vi "SERIAL_Initialize.vi"(1 "navX Device TypeDef":T1={"navX Interface Protocol"=enum."SPI", "navX Interface Protocol TypeDefs"={"SPIDevRef"={"DevStatus"={"status"=FALSE, "code"=0, "source"=""}, "Handle"=0, "Controller"=enum."Controller 1", "SPI Bus"=enum."SPI On-Board, CS0"}, "I2CDevRef"={"DevStatus"={"status"=FALSE, "code"=0, "source"=""}, "Controller"=enum."Controller 1", "Device Address"=0, "Handle"=0, "I2C Bus"=enum."Invalid"}, "SerialPortRef"={"DevStatus"={"status"=FALSE, "code"=0, "source"=""}, "Serial Port Name"=""}}, "navX System Information"={"Board Information"={"WhoAmI (50 | 0x32)"=0, "Board Revision"=0, "Firmware Major Version"=0, "Firmware Minor Version"=0, "NAVX_BOARD_CAPABILITY"={"OMNIMOUNT"=FALSE, "YAW_RESET"=FALSE, "VEL_AND_DISP"=FALSE}, "NAVX_BOARD_YAW_AXIS"={"BOARD_YAW_AXIS_UP"=FALSE, "BOARD_YAW_AXIS"=0}}, "Status"={"Update Rate Hz"=0, "Accelerometer Full-Scale Range"=0, "Gyro Full-Scale Range"=0, "NAVX_OP_STATUS"=0, "NAVX_CAL_STATUS"=0, "NAVX_SELFTEST_STATUS"=0, "NAVX_SENSOR_STATUS"={"MOVING"=FALSE, "YAW_STABLE"=FALSE, "MAG_DISTURBANCE"=FALSE, "ALTITUDE_VALID"=FALSE, "SEALEVEL_PRESS_SET"=FALSE, "FUSED_HEADING_VALID"=FALSE}}, "Offsets"={"Yaw"=0.0, "Quat W"=0.0, "Quat X"=0.0, "Quat Y"=0.0, "Quat Z"=0.0}, "LastSampleTimestamp"=0.0, "LastSampleValid"=FALSE}, "navX Common Information"={"Update Rate (4Hz-60Hz)"=50, "refnum name"="", "error"={"status"=FALSE, "code"=0, "source"=""}, "LastFPGATimestamp"=0.0, "Reboot Detected"=FALSE}, "Serial Protocol Extra"={"Loop VI Refnum"=refnum, "Nav6Mode (YPR)"=enum."Raw"}} {"navX Common Information"."Update Rate (4Hz-60Hz)" min=4 max=60 step=1; "navX System Information"."Status"."NAVX_OP_STATUS" items=["INITIALIZING", "SELFTEST_IN_PROGRESS", "ERROR", "IMU_AUTOCAL_IN_PROGRESS", "NORMAL"]; "navX System Information"."Status"."NAVX_CAL_STATUS" items=["IMU_CAL_STATE_MASK"=3, "IMU_CAL_INPROGRESS"=0, "IMU_CAL_ACCUMULATE"=1, "IMU_CAL_COMPLETE"=2, "MAG_CAL_COMPLETE"=4, "BARO_CAL_COMPLETE"=8]; "navX System Information"."Status"."NAVX_SELFTEST_STATUS" items=["COMPLETE"=80, "GYRO_PASSED"=1, "ACCEL_PASSED"=2, "MAG_PASSED"=4, "BARO_PASSED"=8]; "navX Interface Protocol TypeDefs"."I2CDevRef"."Device Address" format="%.0x"}) -> (0 "navX Device TypeDef":T1={"navX Interface Protocol"=enum."SPI", "navX Interface Protocol TypeDefs"={"SPIDevRef"={"DevStatus"={"status"=FALSE, "code"=0, "source"=""}, "Handle"=0, "Controller"=enum."Controller 1", "SPI Bus"=enum."SPI On-Board, CS0"}, "I2CDevRef"={"DevStatus"={"status"=FALSE, "code"=0, "source"=""}, "Controller"=enum."Controller 1", "Device Address"=0, "Handle"=0, "I2C Bus"=enum."Invalid"}, "SerialPortRef"={"DevStatus"={"status"=FALSE, "code"=0, "source"=""}, "Serial Port Name"=""}}, "navX System Information"={"Board Information"={"WhoAmI (50 | 0x32)"=0, "Board Revision"=0, "Firmware Major Version"=0, "Firmware Minor Version"=0, "NAVX_BOARD_CAPABILITY"={"OMNIMOUNT"=FALSE, "YAW_RESET"=FALSE, "VEL_AND_DISP"=FALSE}, "NAVX_BOARD_YAW_AXIS"={"BOARD_YAW_AXIS_UP"=FALSE, "BOARD_YAW_AXIS"=0}}, "Status"={"Update Rate Hz"=0, "Accelerometer Full-Scale Range"=0, "Gyro Full-Scale Range"=0, "NAVX_OP_STATUS"=0, "NAVX_CAL_STATUS"=0, "NAVX_SELFTEST_STATUS"=0, "NAVX_SENSOR_STATUS"={"MOVING"=FALSE, "YAW_STABLE"=FALSE, "MAG_DISTURBANCE"=FALSE, "ALTITUDE_VALID"=FALSE, "SEALEVEL_PRESS_SET"=FALSE, "FUSED_HEADING_VALID"=FALSE}}, "Offsets"={"Yaw"=0.0, "Quat W"=0.0, "Quat X"=0.0, "Quat Y"=0.0, "Quat Z"=0.0}, "LastSampleTimestamp"=0.0, "LastSampleValid"=FALSE}, "navX Common Information"={"Update Rate (4Hz-60Hz)"=50, "refnum name"="", "error"={"status"=FALSE, "code"=0, "source"=""}, "LastFPGATimestamp"=0.0, "Reboot Detected"=FALSE}, "Serial Protocol Extra"={"Loop VI Refnum"=refnum, "Nav6Mode (YPR)"=enum."Raw"}} {"navX Common Information"."Update Rate (4Hz-60Hz)" min=4 max=60 step=1; "navX System Information"."Status"."NAVX_OP_STATUS" items=["INITIALIZING", "SELFTEST_IN_PROGRESS", "ERROR", "IMU_AUTOCAL_IN_PROGRESS", "NORMAL"]; "navX System Information"."Status"."NAVX_CAL_STATUS" items=["IMU_CAL_STATE_MASK"=3, "IMU_CAL_INPROGRESS"=0, "IMU_CAL_ACCUMULATE"=1, "IMU_CAL_COMPLETE"=2, "MAG_CAL_COMPLETE"=4, "BARO_CAL_COMPLETE"=8]; "navX System Information"."Status"."NAVX_SELFTEST_STATUS" items=["COMPLETE"=80, "GYRO_PASSED"=1, "ACCEL_PASSED"=2, "MAG_PASSED"=4, "BARO_PASSED"=8]; "navX Interface Protocol TypeDefs"."I2CDevRef"."Device Address" format="%.0x"})   [LabVIEW 2014, in "navX-MXP IMU.lvlib"]
uses:
  navX-MXP IMU.lvlib
  COMMON/TypeDefs/navX Device TypeDef.ctl
  COMMON/TypeDefs/Value TypeDefs/navX Interface Protocol.ctl
  <vilib>/Rock Robotics/WPI/SPI/WPI_SPIDevRef.ctl
  <vilib>/Rock Robotics/SystemInterfaces/Typedef/FPGA_TypedefDigitalModule.ctl
  <vilib>/Rock Robotics/SystemInterfaces/spilib/spi_bus.ctl
  <vilib>/Rock Robotics/WPI/I2C/WPI_I2CDevRef.ctl
  <vilib>/Rock Robotics/SystemInterfaces/i2clib/i2c_bus.ctl
  <vilib>/Rock Robotics/WPI/SerialPort/WPI_SerialPortRef.ctl
  COMMON/TypeDefs/Data TypeDefs/navX Board Information.ctl
  COMMON/TypeDefs/Value TypeDefs/navX NAVX_BOARD_CAPABILITY.ctl
  COMMON/TypeDefs/Value TypeDefs/navX NAVX_BOARD_YAW_AXIS.ctl
  COMMON/TypeDefs/Data TypeDefs/navX Status Data.ctl
  COMMON/TypeDefs/Value TypeDefs/navX NAVX_OP_STATUS.ctl
  COMMON/TypeDefs/Value TypeDefs/navX NAVX_CAL_STATUS.ctl
  COMMON/TypeDefs/Value TypeDefs/navX NAVX_SELFTEST_STATUS.ctl
  COMMON/TypeDefs/Value TypeDefs/navX NAVX_SENSOR_STATUS.ctl
  COMMON/TypeDefs/Data TypeDefs/navX Offsets Data.ctl
  COMMON/TypeDefs/Value TypeDefs/navX Update Rate.ctl
  COMMON/TypeDefs/Value TypeDefs/navX Serial Mode.ctl
  COMMON/TypeDefs/Value TypeDefs/navX Device Registers.ctl
  COMMON/TypeDefs/Value TypeDefs/navX NAVX_CAPABILITY_FLAGS.ctl
  <vilib>/Rock Robotics/SystemInterfaces/Utilities/FPGA_UtilitiesRead LocalTime.vi
  COMMON/Util/DataConvert/navX-to-LabVIEW/DecodeRatio.vi
  COMMON/Util/DataConvert/navX-to-LabVIEW/DecodeSignedHundredths.vi
  COMMON/Util/DataConvert/navX-to-LabVIEW/DecodeUInt16.vi
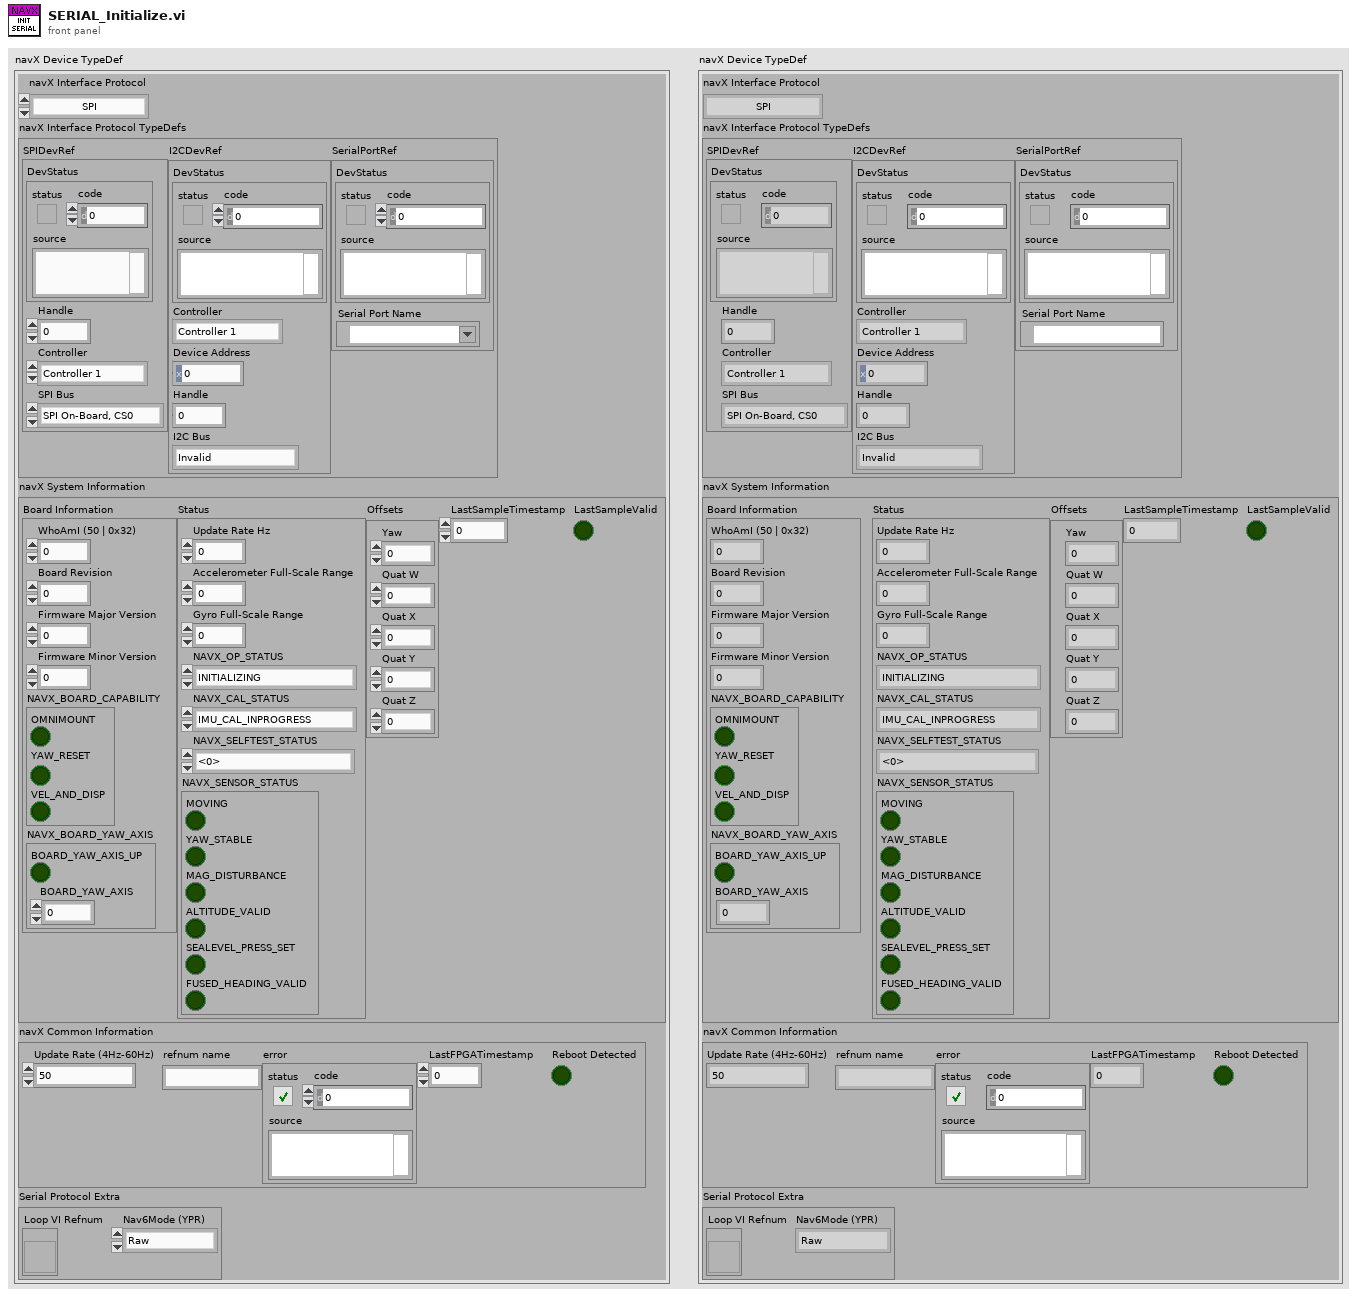
[diagram p1: front panel]
types:
  T1 = typedef "navX-MXP IMU.lvlib/navX Device TypeDef.ctl" = cluster{"navX Interface Protocol":T2, "navX Interface Protocol TypeDefs":cluster{"SPIDevRef":T3, "I2CDevRef":T6, "SerialPortRef":T8}, "navX System Information":cluster{"Board Information":T9, "Status":T12, "Offsets":T17, "LastSampleTimestamp":dbl, "LastSampleValid":bool}, "navX Common Information":cluster{"Update Rate (4Hz-60Hz)":T18, "refnum name":string, "error":errorcluster, "LastFPGATimestamp":dbl, "Reboot Detected":bool}, "Serial Protocol Extra":cluster{"Loop VI Refnum":refnum<vi>, "Nav6Mode (YPR)":T19}}
  T2 = typedef "navX-MXP IMU.lvlib/navX Interface Protocol.ctl" = enum16{"SPI", "I2C", "SERIAL"}
  T3 = typedef "WPI_SPIDevRef.ctl" = cluster{"DevStatus":errorcluster, "Handle":i32, "Controller":T4, "SPI Bus":T5}
  T4 = typedef "FPGA_TypedefDigitalModule.ctl" = enum16{"Controller 1"}
  T5 = typedef "spi_bus.ctl" = enum16{"SPI On-Board, CS0", "SPI On-Board, CS1", "SPI On-Board, CS2", "SPI On-Board, CS3", "SPI MXP", "Invalid"}
  T6 = typedef "WPI_I2CDevRef.ctl" = cluster{"DevStatus":errorcluster, "Controller":T4, "Device Address":u8, "Handle":i32, "I2C Bus":T7}
  T7 = typedef "i2c_bus.ctl" = enum16{"I2C On-Board", "I2C MXP", "Invalid"}
  T8 = typedef "WPI_SerialPortRef.ctl" = cluster{"DevStatus":errorcluster, "Serial Port Name":refnum<visa-resource-name>}
  T9 = typedef "navX-MXP IMU.lvlib/navX Board Information.ctl" = cluster{"WhoAmI (50 | 0x32)":u8, "Board Revision":u8, "Firmware Major Version":u8, "Firmware Minor Version":u8, "NAVX_BOARD_CAPABILITY":T10, "NAVX_BOARD_YAW_AXIS":T11}
  T10 = typedef "navX-MXP IMU.lvlib/navX NAVX_BOARD_CAPABILITY.ctl" = cluster{"OMNIMOUNT":bool, "YAW_RESET":bool, "VEL_AND_DISP":bool}
  T11 = typedef "navX-MXP IMU.lvlib/navX NAVX_BOARD_YAW_AXIS.ctl" = cluster{"BOARD_YAW_AXIS_UP":bool, "BOARD_YAW_AXIS":u8}
  T12 = typedef "navX-MXP IMU.lvlib/navX Status Data.ctl" = cluster{"Update Rate Hz":u8, "Accelerometer Full-Scale Range":u8, "Gyro Full-Scale Range":u16, "NAVX_OP_STATUS":T13, "NAVX_CAL_STATUS":T14, "NAVX_SELFTEST_STATUS":T15, "NAVX_SENSOR_STATUS":T16}
  T13 = typedef "navX-MXP IMU.lvlib/navX NAVX_OP_STATUS.ctl" = u8
  T14 = typedef "navX-MXP IMU.lvlib/navX NAVX_CAL_STATUS.ctl" = u8
  T15 = typedef "navX-MXP IMU.lvlib/navX NAVX_SELFTEST_STATUS.ctl" = u8
  T16 = typedef "navX-MXP IMU.lvlib/navX NAVX_SENSOR_STATUS.ctl" = cluster{"MOVING":bool, "YAW_STABLE":bool, "MAG_DISTURBANCE":bool, "ALTITUDE_VALID":bool, "SEALEVEL_PRESS_SET":bool, "FUSED_HEADING_VALID":bool}
  T17 = typedef "navX-MXP IMU.lvlib/navX Offsets Data.ctl" = cluster{"Yaw":dbl, "Quat W":dbl, "Quat X":dbl, "Quat Y":dbl, "Quat Z":dbl}
  T18 = typedef "navX-MXP IMU.lvlib/navX Update Rate.ctl" = u8
  T19 = typedef "navX-MXP IMU.lvlib/navX Serial Mode.ctl" = enum16{"Raw", "Processed"}
  T20 = typedef "navX-MXP IMU.lvlib/navX Device Registers.ctl" = u8
  T21 = typedef "navX-MXP IMU.lvlib/navX NAVX_CAPABILITY_FLAGS.ctl" = u8
  T22 = cluster{"[0]":dbl, "[1]":dbl, "[2]":dbl, "[3]":dbl, "[4]":dbl}
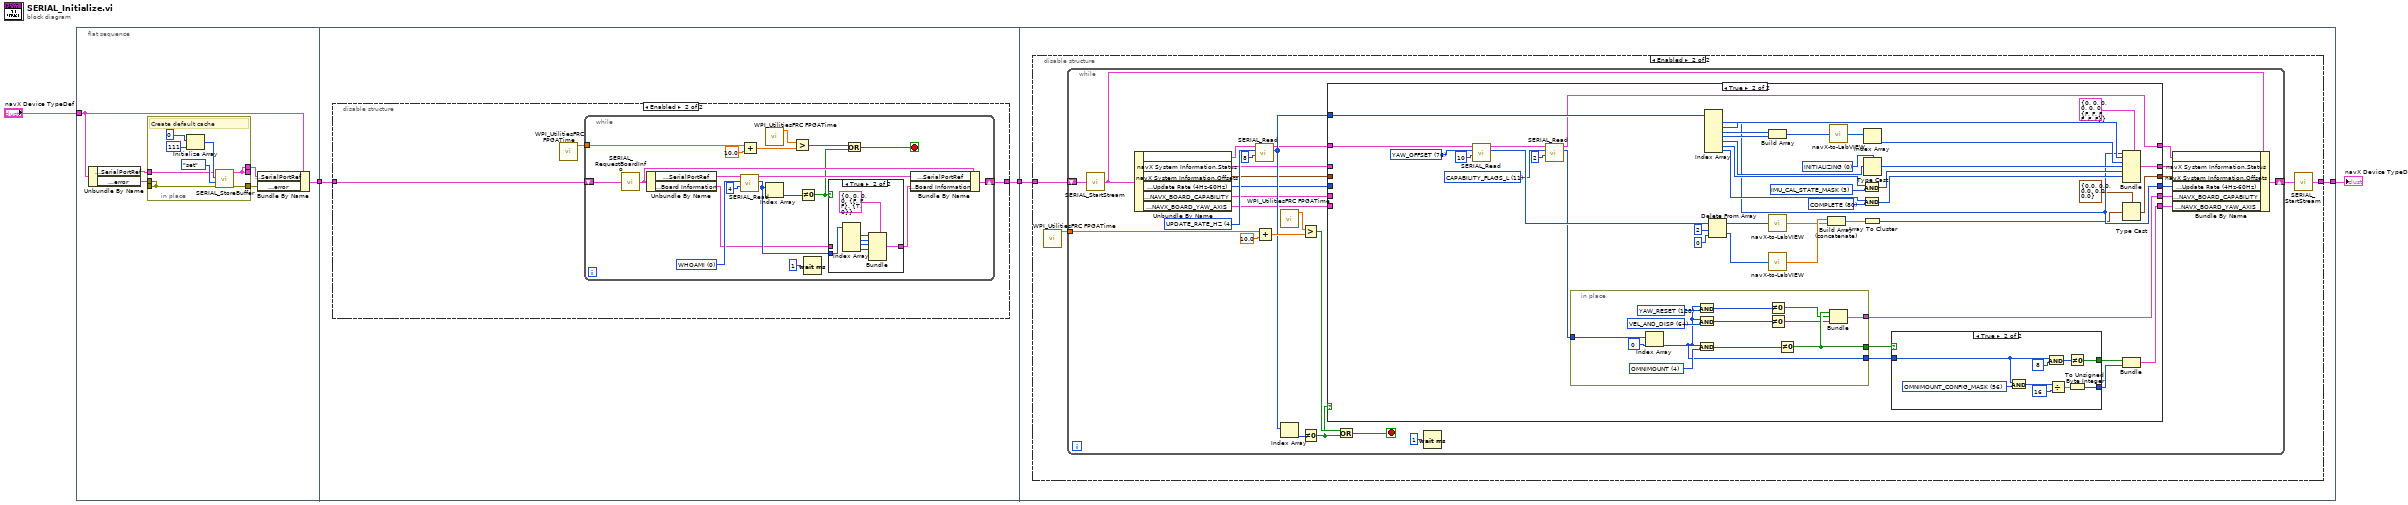
[diagram p0: block diagram]
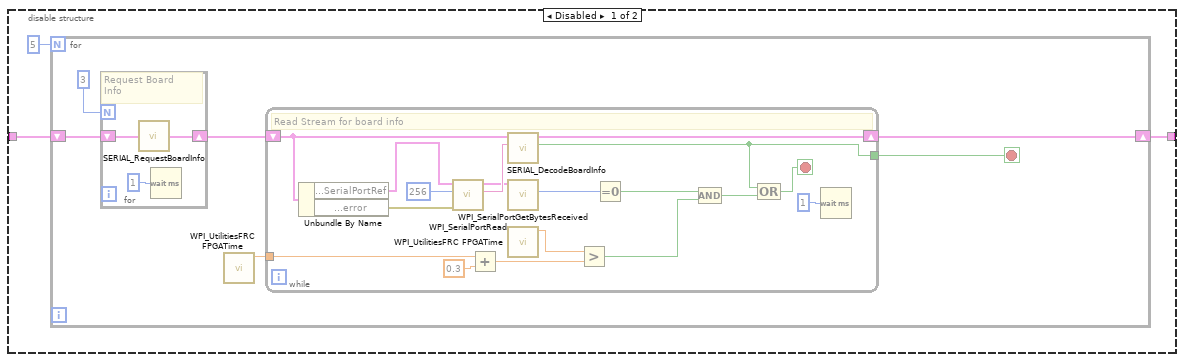
[diagram p2: hidden frame]
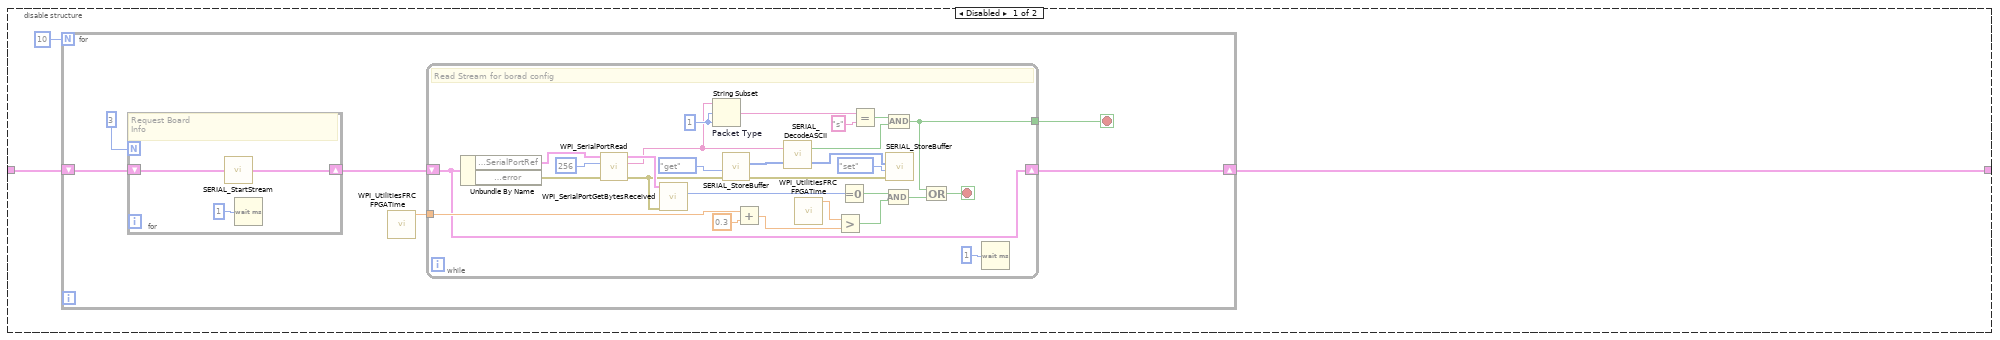
[diagram p4: hidden frame]
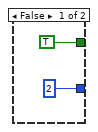
[diagram p6: hidden frame]
diagram:
  n1 = flat-sequence {
    tunnel: "navX Device TypeDef" -> [w6]
    tunnel: [w5] -> w1
    tunnel: [w20] -> w2
    tunnel: w1 -> [w19]
    tunnel: [w81] -> w4
    tunnel: w2 -> [w82]
    frame #0 {
      n2 = Unbundle By Name(w6) -> ("navX Interface Protocol TypeDefs.SerialPortRef"=w10:T8, "navX Common Information.error"=w9:errorcluster)
      n3 = in-place {
        in-place-border: w10 -> [w14]
        in-place-border: [w12] -> _
        in-place-border: [w13] -> w8
        in-place-border: [w11] -> _
        in-place-border: w9 -> [w12]
        in-place-border: [w11] -> w7
        # "Create default cache"
        n4 = Initialize Array(u8 0 ("Received Data"), u8 111 ("hex")) -> (w15:u8[])
        n5 = call "SERIAL_StoreBuffer.vi"("error in (no error)"=w12, "Access Type"=enum16{"set", "get", "delete"}."set", "navX Data"=w15, "SerialPortRef"=w14) -> ("error out"=w13:errorcluster, "SerialPortRef"=w11:T8)  [unwired: 5 in, 1 out]
      }
      n6 = Bundle By Name(cluster=w6, "navX Interface Protocol TypeDefs.SerialPortRef"=w7, "navX Common Information.error"=w8) -> (w5:T1)
    }
    frame #1 {
      n7 = disable-structure shown="Enabled" {
        disable-tunnel: [w23 w52] -> w20
        disable-tunnel: w19 -> [w22 w53]
        frame Disabled {
          n8 = for {
            N: 5 -> [_]
            shift-right: [w25] -> w23
            shift-left: w22 -> [w27]
            stop <- w24 stop-if-true
            n9 = for {
              N: 3 -> [_]
              shift-right: [w31] -> w28
              shift-left: w27 -> [w32]
              # "Request Board\nInfo"
              n10 = call "SERIAL_RequestBoardInfo.vi"("navX Device TypeDef"=w32) -> ("navX Device TypeDef"=w31:T1)
              n11 = Wait (ms)(milliseconds to wait=u32 1) -> ()  [unwired: 1 out]
            }
            n12 = call <vilib>:"WPI_UtilitiesFRC FPGATime.vi"() -> ("FPGA Time"=w26:dbl)  [unwired: 10 in, 1 out]
            n13 = while {
              tunnel: w26 -> [w50]
              shift-right: [w35] -> w25
              shift-left: w28 -> [w41]
              tunnel: [w34] -> w24
              stop <- w36 stop-if-true
              # "Read Stream for board info"
              n14 = Unbundle By Name(w41) -> ("navX Interface Protocol TypeDefs.SerialPortRef"=w43:T8, "navX Common Information.error"=w44:errorcluster)
              n15 = call <vilib>:"WPI_SerialPortRead.vi"("error in (no error)"=w44, "Num Bytes to Read"=u32 256, "SerialPortRef"=w43) -> ("Buffer"=w40:string, "SerialPortRef"=w39:T8)  [unwired: 6 in, 1 out]
              n16 = Add(x=w50, y=0.3) -> (x+y=w47:dbl)
              n17 = call "SERIAL_DecodeBoardInfo.vi"("Buffer"=w40, "navX Device TypeDef"=w41) -> ("Valid?"=w34:bool, "navX Device TypeDef"=w35:T1)  [unwired: 8 in]
              n18 = call <vilib>:"WPI_SerialPortGetBytesReceived.vi"("SerialPortRef"=w39) -> ("Bytes at Port"=w38:u32)  [unwired: 8 in, 2 out]
              n19 = call <vilib>:"WPI_UtilitiesFRC FPGATime.vi"() -> ("FPGA Time"=w48:dbl)  [unwired: 10 in, 1 out]
              n20 = Greater?(x=w48, y=w47) -> (0:w45:bool)
              n21 = Equal To 0?(x=w38) -> (x = 0?=w37:bool)
              n22 = Compound Arithmetic op=AND(w37, w45) -> (w46:bool)
              n23 = Compound Arithmetic op=OR(w34, w46) -> (w36:bool)
              n24 = Wait (ms)(milliseconds to wait=u32 1) -> ()  [unwired: 1 out]
            }
          }
        }
        frame Enabled {
          n25 = call <vilib>:"WPI_UtilitiesFRC FPGATime.vi"() -> ("FPGA Time"=w51:dbl)  [unwired: 10 in, 1 out]
          n26 = while {
            shift-right: [w60] -> w52
            shift-left: w53 -> [w72]
            tunnel: w51 -> [w67]
            stop <- w66 stop-if-true
            w58 = T20 0 items=["WHOAMI"=0, "HW_REV"=1, "FW_VER_MAJOR"=2, "FW_VER_MINOR"=3, "UPDATE_RATE_HZ"=4, "ACCEL_FSR_G"=5, "GYRO_FSR_DPS"=6, "OP_STATUS"=8, "CAL_STATUS"=9, "SELFTEST_STATUS"=10, "CAPABILITY_FLAGS_L"=11, "CAPABILITY_FLAGS_H"=12, "SENSOR_STATUS"=16, "TIMESTAMP"=18, "YAW"=22, "PITCH"=24, "ROLL"=26, "HEADING"=28, "FUSED_HEADING"=30, "ALTITUDE_I"=32, "ALTITUDE_D"=34, "LINERA_ACC_X"=36, "LINERA_ACC_Y"=38, "LINERA_ACC_Z"=40, "QUAT_W"=42, "QUAT_X"=44, "QUAT_Y"=46, "QUAT_Z"=48, "MPU_TEMP_C"=50, "GYRO_X"=52, "GYRO_Y"=54, "GYRO_Z"=56, "ACC_X"=58, "ACC_Y"=60, "ACC_Z"=62, "MAG_X"=64, "MAG_Y"=66, "MAG_Z"=68, "PRESSURE_I"=70, "PRESSURE_D"=72, "PRESSURE_TEMP"=74, "YAW_OFFSET"=76, "QUAT_OFFSET_W"=78, "QUAT_OFFSET_X"=80, "QUAT_OFFSET_Y"=82, "QUAT_OFFSET_Z"=84, "INTEGRATION_CONTROL"=86, "VELOCITY_X"=88, "VELOCITY_Y"=92, "VELOCITY_Z"=96, "DISPLACMENT_X"=100, "DISPLACMENT_Y"=104, "DISPLACEMENT_Z"=108] ("Device Register")
            n27 = call "SERIAL_RequestBoardInfo.vi"("navX Device TypeDef"=w72) -> ("navX Device TypeDef"=w64:T1)
            n28 = Unbundle By Name(w64) -> ("navX Interface Protocol TypeDefs.SerialPortRef"=w63:T8, "navX System Information.Board Information"=w54:T9)
            n29 = call "SERIAL_Read.vi"("Read Size"=u8 4, "Device Register"=w58, "SerialPortRef"=w63) -> ("navX Data"=w57:u8[], "SerialPortRef"=w62:T8)  [unwired: 6 in, 1 out]
            n30 = Add(x=w67, y=10.0) -> (x+y=w69:dbl)
            n31 = call <vilib>:"WPI_UtilitiesFRC FPGATime.vi"() -> ("FPGA Time"=w70:dbl)  [unwired: 10 in, 1 out]
            n32 = Index Array(array=w57) -> (element=w61:u8)  [unwired: 1 in]
            n33 = Greater?(x=w70, y=w69) -> (0:w65:bool)
            n34 = Not Equal To 0?(x=w61) -> (x != 0?=w55:bool)
            n35 = Wait (ms)(milliseconds to wait=u32 1) -> ()  [unwired: 1 out]
            n36 = case shown="True" w55 {
              tunnel: w57 -> [_ w80]
              tunnel: [w73 w79] -> w56
              tunnel: w54 -> [w73 _]
              frame False {
              }
              frame True {
                n37 = Index Array(array=w80) -> (element #1=w77:u8, element #2=w76:u8, element #3=w75:u8, element #4=w74:u8)  [unwired: 4 in]
                n38 = Bundle(cluster=T9 {"WhoAmI (50 | 0x32)"=0, "Board Revision"=0, "Firmware Major Version"=0, "Firmware Minor Version"=0, "NAVX_BOARD_CAPABILITY"={"OMNIMOUNT"=FALSE, "YAW_RESET"=FALSE, "VEL_AND_DISP"=FALSE}, "NAVX_BOARD_YAW_AXIS"={"BOARD_YAW_AXIS_UP"=TRUE, "BOARD_YAW_AXIS"=0}} ("Board Information"), "WhoAmI (50 | 0x32)"=w77, "Board Revision"=w76, "Firmware Major Version"=w75, "Firmware Minor Version"=w74) -> (w79:T9)  [unwired: 2 in]
              }
            }
            n39 = Or(x=w65, y=w55) -> (x .or. y?=w66:bool)
            n40 = Bundle By Name(cluster=w64, "navX Interface Protocol TypeDefs.SerialPortRef"=w62, "navX System Information.Board Information"=w56) -> (w60:T1)
          }
        }
      }
    }
    frame #2 {
      n41 = disable-structure shown="Enabled" {
        disable-tunnel: w82 -> [w84 w126]
        disable-tunnel: [w83 w123] -> w81
        frame Disabled {
          n42 = for {
            N: 10 -> [_]
            shift-right: [w87] -> w83
            shift-left: w84 -> [w89]
            stop <- w86 stop-if-true
            n43 = for {
              N: 3 -> [_]
              shift-right: [w92] -> w90
              shift-left: w89 -> [w93]
              # "Request Board\nInfo"
              n44 = call "SERIAL_StartStream.vi"("navX Device TypeDef"=w93) -> ("navX Device TypeDef"=w92:T1)
              n45 = Wait (ms)(milliseconds to wait=u32 1) -> ()  [unwired: 1 out]
            }
            n46 = call <vilib>:"WPI_UtilitiesFRC FPGATime.vi"() -> ("FPGA Time"=w88:dbl)  [unwired: 10 in, 1 out]
            n47 = while {
              tunnel: w88 -> [w122]
              shift-right: [w108] -> w87
              shift-left: w90 -> [w108]
              tunnel: [w97] -> w86
              stop <- w110 stop-if-true
              w105 = 1 ("offset (0)")
              # "Read Stream for borad config"
              n48 = Unbundle By Name(w108) -> ("navX Interface Protocol TypeDefs.SerialPortRef"=w115:T8, "navX Common Information.error"=w116:errorcluster)
              n49 = call <vilib>:"WPI_SerialPortRead.vi"("error in (no error)"=w116, "Num Bytes to Read"=u32 256, "SerialPortRef"=w115) -> ("error out"=w95:errorcluster, "Buffer"=w104:string, "SerialPortRef"=w113:T8)  [unwired: 6 in]
              n50 = call <vilib>:"WPI_SerialPortGetBytesReceived.vi"("error in (no error)"=w95, "SerialPortRef"=w113) -> ("Bytes at Port"=w112:u32)  [unwired: 7 in, 2 out]
              n51 = String Subset "Packet Type"(string=w104, offset (0)=w105, length (rest)=w105) -> (substring=w103:string)
              n52 = call "SERIAL_StoreBuffer.vi"("error in (no error)"=w95, "Access Type"=enum16{"set", "get", "delete"}."get") -> ("error out"=w96:errorcluster, "navX Data"=w107:u8[])  [unwired: 7 in, 1 out]
              n53 = Add(x=w122, y=0.3) -> (x+y=w119:dbl)
              n54 = call "SERIAL_DecodeASCII.vi"("navX Data"=w107, "Buffer"=w104) -> ("navX Data"=w100:u8[], "Valid?"=w98:bool)
              n55 = call <vilib>:"WPI_UtilitiesFRC FPGATime.vi"() -> ("FPGA Time"=w120:dbl)  [unwired: 10 in, 1 out]
              n56 = Greater?(x=w120, y=w119) -> (0:w117:bool)
              n57 = Equal To 0?(x=w112) -> (x = 0?=w111:bool)
              n58 = Equal?(x=w103, y="s") -> (x = y?=w99:bool)
              n59 = call "SERIAL_StoreBuffer.vi"("error in (no error)"=w96, "Access Type"=enum16{"set", "get", "delete"}."set", "navX Data"=w100) -> ()  [unwired: 6 in, 3 out]
              n60 = Compound Arithmetic op=AND(w111, w117) -> (w118:bool)
              n61 = Compound Arithmetic op=AND(w99, w98) -> (w97:bool)
              n62 = Compound Arithmetic op=OR(w97, w118) -> (w110:bool)
              n63 = Wait (ms)(milliseconds to wait=u32 1) -> ()  [unwired: 1 out]
            }
          }
        }
        frame Enabled {
          n64 = call <vilib>:"WPI_UtilitiesFRC FPGATime.vi"() -> ("FPGA Time"=w125:dbl)  [unwired: 10 in, 1 out]
          n65 = while {
            shift-right: [w151] -> w124
            shift-left: w126 -> [w153]
            tunnel: w125 -> [w146]
            stop <- w144 stop-if-true
            w143 = T20 4 items=["WHOAMI"=0, "HW_REV"=1, "FW_VER_MAJOR"=2, "FW_VER_MINOR"=3, "UPDATE_RATE_HZ"=4, "ACCEL_FSR_G"=5, "GYRO_FSR_DPS"=6, "OP_STATUS"=8, "CAL_STATUS"=9, "SELFTEST_STATUS"=10, "CAPABILITY_FLAGS_L"=11, "CAPABILITY_FLAGS_H"=12, "SENSOR_STATUS"=16, "TIMESTAMP"=18, "YAW"=22, "PITCH"=24, "ROLL"=26, "HEADING"=28, "FUSED_HEADING"=30, "ALTITUDE_I"=32, "ALTITUDE_D"=34, "LINERA_ACC_X"=36, "LINERA_ACC_Y"=38, "LINERA_ACC_Z"=40, "QUAT_W"=42, "QUAT_X"=44, "QUAT_Y"=46, "QUAT_Z"=48, "MPU_TEMP_C"=50, "GYRO_X"=52, "GYRO_Y"=54, "GYRO_Z"=56, "ACC_X"=58, "ACC_Y"=60, "ACC_Z"=62, "MAG_X"=64, "MAG_Y"=66, "MAG_Z"=68, "PRESSURE_I"=70, "PRESSURE_D"=72, "PRESSURE_TEMP"=74, "YAW_OFFSET"=76, "QUAT_OFFSET_W"=78, "QUAT_OFFSET_X"=80, "QUAT_OFFSET_Y"=82, "QUAT_OFFSET_Z"=84, "INTEGRATION_CONTROL"=86, "VELOCITY_X"=88, "VELOCITY_Y"=92, "VELOCITY_Z"=96, "DISPLACMENT_X"=100, "DISPLACMENT_Y"=104, "DISPLACEMENT_Z"=108] ("Device Register")
            n66 = call "SERIAL_StartStream.vi"("navX Device TypeDef"=w153) -> ("navX Device TypeDef"=w152:T1)
            n67 = Unbundle By Name(w152) -> ("navX Interface Protocol TypeDefs.SerialPortRef"=w150:T8, "navX System Information.Status"=w138:T12, "navX System Information.Offsets"=w136:T17, "navX Common Information.Update Rate (4Hz-60Hz)"=w133:T18, "navX System Information.Board Information.NAVX_BOARD_CAPABILITY"=w128:T10, "navX System Information.Board Information.NAVX_BOARD_YAW_AXIS"=w127:T11)
            n68 = call "SERIAL_Read.vi"("Read Size"=u8 8, "Device Register"=w143, "SerialPortRef"=w150) -> ("navX Data"=w139:u8[], "SerialPortRef"=w132:T8)  [unwired: 6 in, 1 out]
            n69 = Add(x=w146, y=10.0) -> (x+y=w148:dbl)
            n70 = call <vilib>:"WPI_UtilitiesFRC FPGATime.vi"() -> ("FPGA Time"=w147:dbl)  [unwired: 10 in, 1 out]
            n71 = Index Array(array=w139) -> (element=w141:u8)  [unwired: 1 in]
            n72 = Greater?(x=w147, y=w148) -> (0:w149:bool)
            n73 = Not Equal To 0?(x=w141) -> (x != 0?=w140:bool)
            n74 = case shown="True" w140 {
              tunnel: w139 -> [_ w204]
              tunnel: [w160 w187] -> w137
              tunnel: w138 -> [w160 _]
              tunnel: w136 -> [w159 _]
              tunnel: [w159 w173] -> w135
              tunnel: [w158 w186] -> w134
              tunnel: w133 -> [w158 _]
              tunnel: w132 -> [w157 w167]
              tunnel: [w157 w165] -> w131
              tunnel: [w155 w162] -> w130
              tunnel: [w156 w161] -> w129
              tunnel: w128 -> [w156 _]
              tunnel: w127 -> [w155 _]
              frame False {
              }
              frame True {
                w172 = T20 11 items=["WHOAMI"=0, "HW_REV"=1, "FW_VER_MAJOR"=2, "FW_VER_MINOR"=3, "UPDATE_RATE_HZ"=4, "ACCEL_FSR_G"=5, "GYRO_FSR_DPS"=6, "OP_STATUS"=8, "CAL_STATUS"=9, "SELFTEST_STATUS"=10, "CAPABILITY_FLAGS_L"=11, "CAPABILITY_FLAGS_H"=12, "SENSOR_STATUS"=16, "TIMESTAMP"=18, "YAW"=22, "PITCH"=24, "ROLL"=26, "HEADING"=28, "FUSED_HEADING"=30, "ALTITUDE_I"=32, "ALTITUDE_D"=34, "LINERA_ACC_X"=36, "LINERA_ACC_Y"=38, "LINERA_ACC_Z"=40, "QUAT_W"=42, "QUAT_X"=44, "QUAT_Y"=46, "QUAT_Z"=48, "MPU_TEMP_C"=50, "GYRO_X"=52, "GYRO_Y"=54, "GYRO_Z"=56, "ACC_X"=58, "ACC_Y"=60, "ACC_Z"=62, "MAG_X"=64, "MAG_Y"=66, "MAG_Z"=68, "PRESSURE_I"=70, "PRESSURE_D"=72, "PRESSURE_TEMP"=74, "YAW_OFFSET"=76, "QUAT_OFFSET_W"=78, "QUAT_OFFSET_X"=80, "QUAT_OFFSET_Y"=82, "QUAT_OFFSET_Z"=84, "INTEGRATION_CONTROL"=86, "VELOCITY_X"=88, "VELOCITY_Y"=92, "VELOCITY_Z"=96, "DISPLACMENT_X"=100, "DISPLACMENT_Y"=104, "DISPLACEMENT_Z"=108] ("Device Register")
                w184 = T20 76 items=["WHOAMI"=0, "HW_REV"=1, "FW_VER_MAJOR"=2, "FW_VER_MINOR"=3, "UPDATE_RATE_HZ"=4, "ACCEL_FSR_G"=5, "GYRO_FSR_DPS"=6, "OP_STATUS"=8, "CAL_STATUS"=9, "SELFTEST_STATUS"=10, "CAPABILITY_FLAGS_L"=11, "CAPABILITY_FLAGS_H"=12, "SENSOR_STATUS"=16, "TIMESTAMP"=18, "YAW"=22, "PITCH"=24, "ROLL"=26, "HEADING"=28, "FUSED_HEADING"=30, "ALTITUDE_I"=32, "ALTITUDE_D"=34, "LINERA_ACC_X"=36, "LINERA_ACC_Y"=38, "LINERA_ACC_Z"=40, "QUAT_W"=42, "QUAT_X"=44, "QUAT_Y"=46, "QUAT_Z"=48, "MPU_TEMP_C"=50, "GYRO_X"=52, "GYRO_Y"=54, "GYRO_Z"=56, "ACC_X"=58, "ACC_Y"=60, "ACC_Z"=62, "MAG_X"=64, "MAG_Y"=66, "MAG_Z"=68, "PRESSURE_I"=70, "PRESSURE_D"=72, "PRESSURE_TEMP"=74, "YAW_OFFSET"=76, "QUAT_OFFSET_W"=78, "QUAT_OFFSET_X"=80, "QUAT_OFFSET_Y"=82, "QUAT_OFFSET_Z"=84, "INTEGRATION_CONTROL"=86, "VELOCITY_X"=88, "VELOCITY_Y"=92, "VELOCITY_Z"=96, "DISPLACMENT_X"=100, "DISPLACMENT_Y"=104, "DISPLACEMENT_Z"=108] ("Device Register")
                w190 = T15 80 items=["COMPLETE"=80, "GYRO_PASSED"=1, "ACCEL_PASSED"=2, "MAG_PASSED"=4, "BARO_PASSED"=8] ("NAVX_SELFTEST_STATUS")
                w193 = T14 3 items=["IMU_CAL_STATE_MASK"=3, "IMU_CAL_INPROGRESS"=0, "IMU_CAL_ACCUMULATE"=1, "IMU_CAL_COMPLETE"=2, "MAG_CAL_COMPLETE"=4, "BARO_CAL_COMPLETE"=8] ("NAVX_CAL_STATUS")
                w195 = T13 0 items=["INITIALIZING", "SELFTEST_IN_PROGRESS", "ERROR", "IMU_AUTOCAL_IN_PROGRESS", "NORMAL"] ("NAVX_OP_STATUS")
                n75 = call "SERIAL_Read.vi"("Read Size"=u8 10, "Device Register"=w184, "SerialPortRef"=w167) -> ("navX Data"=w181:u8[], "SerialPortRef"=w166:T8)  [unwired: 6 in, 1 out]
                n76 = call "SERIAL_Read.vi"("Read Size"=u8 2, "Device Register"=w172, "SerialPortRef"=w166) -> ("navX Data"=w168:u8[], "SerialPortRef"=w165:T8)  [unwired: 6 in, 1 out]
                n77 = in-place {
                  in-place-border: w168 -> [w217]
                  in-place-border: [w214] -> w170
                  in-place-border: [w206] -> w169
                  in-place-border: [w205] -> w161
                  w208 = T21 64 items=["OMNIMOUNT"=4, "VEL_AND_DISP "=64, "YAW_RESET"=128, "OMNIMOUNT_CONFIG_MASK"=56] ("NAVX_CAPABILITY_FLAG")
                  w212 = T21 128 items=["OMNIMOUNT"=4, "VEL_AND_DISP "=64, "YAW_RESET"=128, "OMNIMOUNT_CONFIG_MASK"=56] ("NAVX_CAPABILITY_FLAG")
                  w213 = T21 4 items=["OMNIMOUNT"=4, "VEL_AND_DISP "=64, "YAW_RESET"=128, "OMNIMOUNT_CONFIG_MASK"=56] ("NAVX_CAPABILITY_FLAG")
                  n78 = Index Array(array=w217, index=u8 0 ("Read Size")) -> (element=w206:u8)
                  n79 = And(x=w206, y=w212) -> (x .and. y?=w211:T21)
                  n80 = And(x=w206, y=w208) -> (x .and. y?=w209:T21)
                  n81 = And(x=w206, y=w213) -> (x .and. y?=w215:T21)
                  n82 = Not Equal To 0?(x=w211) -> (x != 0?=w210:bool)
                  n83 = Not Equal To 0?(x=w209) -> (x != 0?=w207:bool)
                  n84 = Not Equal To 0?(x=w215) -> (x != 0?=w214:bool)
                  n85 = Bundle(w214, w210, w207) -> (w205:cluster{bool, bool, bool})  [unwired: 1 in]
                }
                n86 = Index Array(array=w204) -> (element #1=w186:u8, element #2=w202:u8, element #3=w201:u8, element #4=w200:u8, element #5=w196:u8, element #6=w192:u8, element #7=w189:u8)  [unwired: 7 in]
                n87 = Delete From Array(array=w181, length=2, index=0) -> (deleted portion=w180:u8[], array with subset deleted=w179:u8[])
                n88 = Build Array(w201, w200) -> (w199:u8[])
                n89 = call-poly "navX-to-LabVIEW.vi"("Data In"=w179) -> ("Data Out"=w177:dbl[])
                n90 = call-poly "navX-to-LabVIEW.vi"("Data In"=w180) -> ("Data Out"=w178:dbl[])
                n91 = Build Array (concatenate)(w178, w177) -> (w176:dbl[])
                n92 = call-poly "navX-to-LabVIEW.vi"("Data In"=w199) -> ("Data Out"=w198:u16[])
                n93 = And(x=w192, y=w193) -> (x .and. y?=w191:T14)
                n94 = And(x=w189, y=w190) -> (x .and. y?=w188:T15)
                n95 = Array To Cluster(array=w176) -> (cluster=w175:T22)
                n96 = Index Array(array=w198) -> (element=w197:u16)  [unwired: 1 in]
                n97 = Type Cast(type=w195, x=w196) -> (*(type *) &x=w194:T13)
                n98 = case shown="True" w170 {
                  tunnel: [TRUE w226] -> w164
                  tunnel: [u8 2 w220] -> w163
                  tunnel: w169 -> [_ w224]
                  frame False {
                  }
                  frame True {
                    w225 = T21 56 items=["OMNIMOUNT"=4, "VEL_AND_DISP "=64, "YAW_RESET"=128, "OMNIMOUNT_CONFIG_MASK"=56] ("NAVX_CAPABILITY_FLAG")
                    n99 = And(x=w224, y=w225) -> (x .and. y?=w223:T21)
                    n100 = And(x=w224, y=u8 8 ("Read Size")) -> (x .and. y?=w227:u8)
                    n101 = Divide(x=w223, y=u8 16 ("Read Size")) -> (x/y=w221:dbl)
                    n102 = Not Equal To 0?(x=w227) -> (x != 0?=w226:bool)
                    n103 = To Unsigned Byte Integer(number=w221) -> (unsigned 8bit integer=w220:u8)
                  }
                }
                n104 = Bundle(cluster=T12 {"Update Rate Hz"=0, "Accelerometer Full-Scale Range"=0, "Gyro Full-Scale Range"=0, "NAVX_OP_STATUS"=0, "NAVX_CAL_STATUS"=0, "NAVX_SELFTEST_STATUS"=0, "NAVX_SENSOR_STATUS"={"MOVING"=FALSE, "YAW_STABLE"=FALSE, "MAG_DISTURBANCE"=FALSE, "ALTITUDE_VALID"=FALSE, "SEALEVEL_PRESS_SET"=FALSE, "FUSED_HEADING_VALID"=FALSE}} ("Status"), "Update Rate Hz"=w186, "Accelerometer Full-Scale Range"=w202, "Gyro Full-Scale Range"=w197, "NAVX_OP_STATUS"=w194, "NAVX_CAL_STATUS"=w191, "NAVX_SELFTEST_STATUS"=w188) -> (w187:T12)  [unwired: 1 in]
                n105 = Type Cast(type=T17 {"Yaw"=0.0, "Quat W"=0.0, "Quat X"=0.0, "Quat Y"=0.0, "Quat Z"=0.0} ("Offsets"), x=w175) -> (*(type *) &x=w173:T17)
                n106 = Bundle(w164, w163) -> (w162:cluster{bool, u8})  [unwired: 1 in]
              }
            }
            n107 = Or(x=w149, y=w140) -> (x .or. y?=w144:bool)
            n108 = Wait (ms)(milliseconds to wait=u32 1) -> ()  [unwired: 1 out]
            n109 = Bundle By Name(cluster=w152, "navX Interface Protocol TypeDefs.SerialPortRef"=w131, "navX System Information.Status"=w137, "navX System Information.Offsets"=w135, "navX Common Information.Update Rate (4Hz-60Hz)"=w134, "navX System Information.Board Information.NAVX_BOARD_CAPABILITY"=w129, "navX System Information.Board Information.NAVX_BOARD_YAW_AXIS"=w130) -> (w151:T1)
          }
          n110 = call "SERIAL_StartStream.vi"("navX Device TypeDef"=w124) -> ("navX Device TypeDef"=w123:T1)
        }
      }
    }
  }
  "navX Device TypeDef" <- w4
